vi "validate key value pair.vi"(8 "error in":errorcluster, 9 "value":string, 10 "key":string, 11 "Watchdog configuration in":refnum<class "Watchdog configuration.lvclass">) -> (0 "error out":errorcluster, 3 "Watchdog configuration out":refnum<class "Watchdog configuration.lvclass">)   [LabVIEW 2013, in "Watchdog configuration.lvclass"]
uses:
  Watchdog configuration.lvclass
  <vilib>/NI/Tag Bus Data Framework/fixed module parent/module/configuration/fixed channel configuration.lvclass
  <vilib>/NI/Configuration Framework/NISE_CEF_TreeControl.lvlib
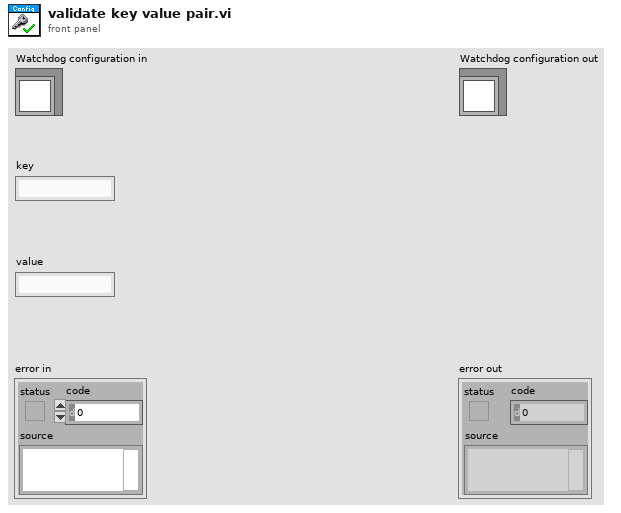
[diagram p1: front panel]
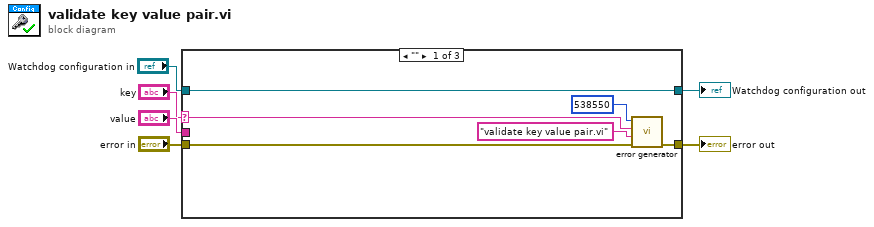
[diagram p0: block diagram]
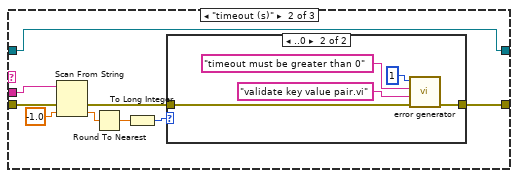
[diagram p2: hidden frame]
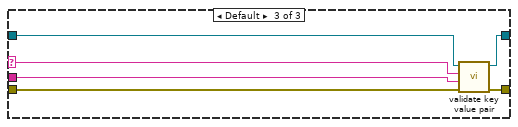
[diagram p4: hidden frame]
diagram:
  n1 = case shown="\"\"" "key" {
    selector: "key" -> [w9 _ w28]
    tunnel: [w7 w21 w33] -> w6
    tunnel: [w12 w19 w32] -> w5
    tunnel: "error in" -> [w8 w20 w31]
    tunnel: "value" -> [_ w17 w30]
    tunnel: "Watchdog configuration in" -> [w12 w19 w29]
    frame "" {
      n2 = call <vilib>:"error generator.vi"("error in"=w8, "source"="validate key value pair.vi", "append error message"=w9, "error code (0)"=538550) -> ("error out"=w7:errorcluster)  [unwired: 5 in]
    }
    frame "timeout (s)" {
      n3 = Scan From String(input string=w17, error in=w20, default 1=-1.0 ("default value 1")) -> (error out=w18:errorcluster, output 1=w15:dbl)  [unwired: 2 in, 2 out]
      n4 = Round To Nearest(number=w15) -> (nearest integer value=w14:dbl)
      n5 = To Long Integer(number=w14) -> (32bit integer=w13:i32)
      n6 = case shown="..0" w13 {
        tunnel: [w22 w26] -> w21
        tunnel: w18 -> [w22 w24]
        frame Default {
        }
        frame ..0 {
          n7 = call <vilib>:"error generator.vi"("error in"=w24, "source"="validate key value pair.vi", "append error message"="timeout must be greater than 0", "error code (0)"=1) -> ("error out"=w26:errorcluster)  [unwired: 5 in]
        }
      }
    }
    frame Default {
      n8 = call-parent "validate key value pair.vi"("error in"=w31, "value"=w30, "key"=w28, "fixed channel configuration in"=w29) -> ("error out"=w33:errorcluster, "fixed channel configuration out"=w32:refnum<class "Watchdog configuration.lvclass">)  [unwired: 6 in]
    }
  }
  "error out" <- w6
  "Watchdog configuration out" <- w5
